vi "Clear Reference.vi"(8 "error in (no error)":errorcluster, 11 "Class Reference Control in":refnum<class "Class Reference Control.lvclass">) -> (0 "error out":errorcluster, 3 "Class Reference Control out":refnum<class "Class Reference Control.lvclass">)   [LabVIEW 2016, in "Class Reference Control.lvclass"]
uses:
  Class Reference Control.lvclass
  Class Reference Control.lvclass/Class Reference Control.ctl
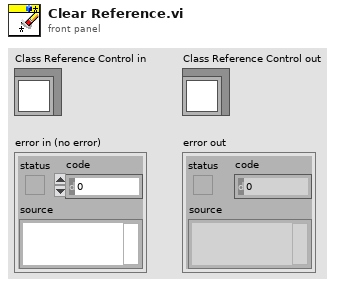
[diagram p1: front panel]
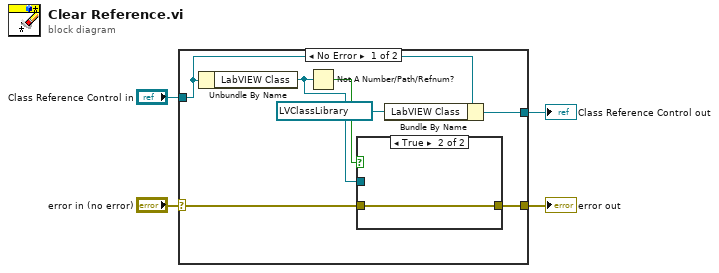
[diagram p0: block diagram]
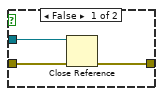
[diagram p2: hidden frame]
diagram:
  n1 = case shown="No Error" "error in (no error)" {
    selector: "error in (no error)" -> [w9 w17]
    tunnel: [w8 w17] -> w1
    tunnel: [w6 w16] -> w2
    tunnel: "Class Reference Control in" -> [w7 w16]
    frame No Error {
      n2 = Unbundle By Name(w7) -> ("LabVIEW Class"=w10:refnum<vi>)
      n3 = Not A Number/Path/Refnum?(number/path/refnum=w10) -> (NaN/Path/Refnum?=w11:bool)
      n4 = case shown="True" w11 {
        tunnel: w10 -> [w14 _]
        tunnel: w9 -> [w13 w15]
        tunnel: [w12 w15] -> w8
        frame False {
          n5 = Close Reference(reference=w14, error in (no error)=w13) -> (error out=w12:errorcluster)
        }
        frame True {
        }
      }
      n6 = Bundle By Name(cluster=w7, "LabVIEW Class"=refnum<vi> refnum) -> (w6:refnum<class "Class Reference Control.lvclass">)
    }
    frame Error {
    }
  }
  "error out" <- w1
  "Class Reference Control out" <- w2
